vi "fpga_globals.vi"() -> ()   [LabVIEW 2014]
panel:
  in  "Output enable":bool[](array[boolean])=[FALSE, FALSE, FALSE, FALSE, FALSE, FALSE, FALSE, FALSE]
  in  "I2C Exit on Empty":bool
  # "If true, causes the I2C bus controllers to exit  as soon as their command FIFOs empty out."
  # "Enable individual timer outputs.  We disable all timers when we shut down to prevent overdriving the LEDs, and we disable individual lights for ASAP testing."
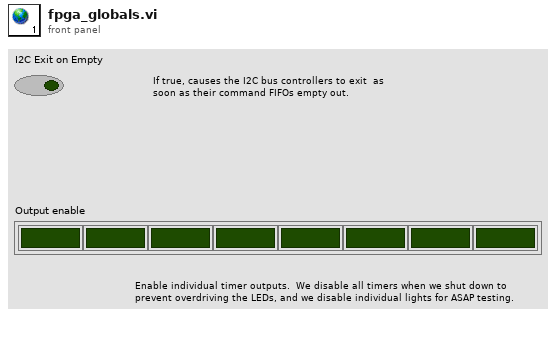
[diagram p1: front panel]
diagram:
